vi "KE6485GUI.panel.vi"() -> ()   [LabVIEW 2014, in "KE6485GUI.lvlib"]
doc: "example GUI for a class inherited from the DeviceBaseGUI\n\nauthor: Dietrich Beck, GSI\nlicense: GPL"
uses:
  KE6485GUI.lvlib
  CSlibraries-extern/DimLVEvent/DimIndicators/DimIndicators.numericType.ctl
  CSlibraries-extern/DimLVEvent/LVDimInterface/LVDimInterface.dim service type.ctl
  <vilib>/Utility/file.llb/Write To Spreadsheet File (DBL).vi
  CS_Core/CSSystem/CoreLib/CoreLib.byte array 2 string.vi
  CS_Core/CSSystem/CoreLib/CoreLib.lvlib
  CS_Core/CSObj/CSObj.lvlib
  CS_Core/GUIs/GOGUserGUIs/DeviceBaseGUI/DeviceBaseGUI.lvlib
  CSlibraries-extern/DimLVEvent/DimIndicators/DimIndicators.lvlib
  CS_Core/CSSystem/CSSystemLib/CSSystemLib.lvlib
  CS_Core/BaseProcess/BaseProcess.lvlib
  CSlibraries-extern/DimLVEvent/LVDimInterface/LVDimInterface.lvlib
panel:
  out "Remaning time":string
  out "running?":bool
  out "ActDimensions":i16
  out "SActStep":i32
  out "SNofSteps":i32
  out "ScanValuesArray":dbl[](array[numeric])
  out "ScanNamesArray":string[](array[string])
  out "size(s)":i32
  in  "Scanner_Finished":T1
  out "DIM Notifier loop":i32
  in  "Free Delay (s)":dbl=1.0
  in  "Data points":u32
  in  "Free Run?":bool
  in  "Save Path":path
  in  "Save button":bool
  in  "Clear Button":bool
  out "actPPG":string
  out "actScanner":string
  out "actSequencer":string
  in  "actValueLink":T1 caption="dic_service_numeric"
  out "Busy":bool
  out "Logger String":string
  out "Progress bar":u8(slide) scale=0.0..100.0
  in  "Stop Scan button":bool
  in  "Pause Scan button":bool
  in  "Start Scan button":bool
  in  "Configure Scan button":bool
  out "chart":cluster{dbl, "data":dbl}[](graph)
  out "loop counter":i32
  out "error out":errorcluster
  in  "error in (no error)":errorcluster
  in  "object ref":refnum<vi>
  # "Scan control"
  # "Plot control"
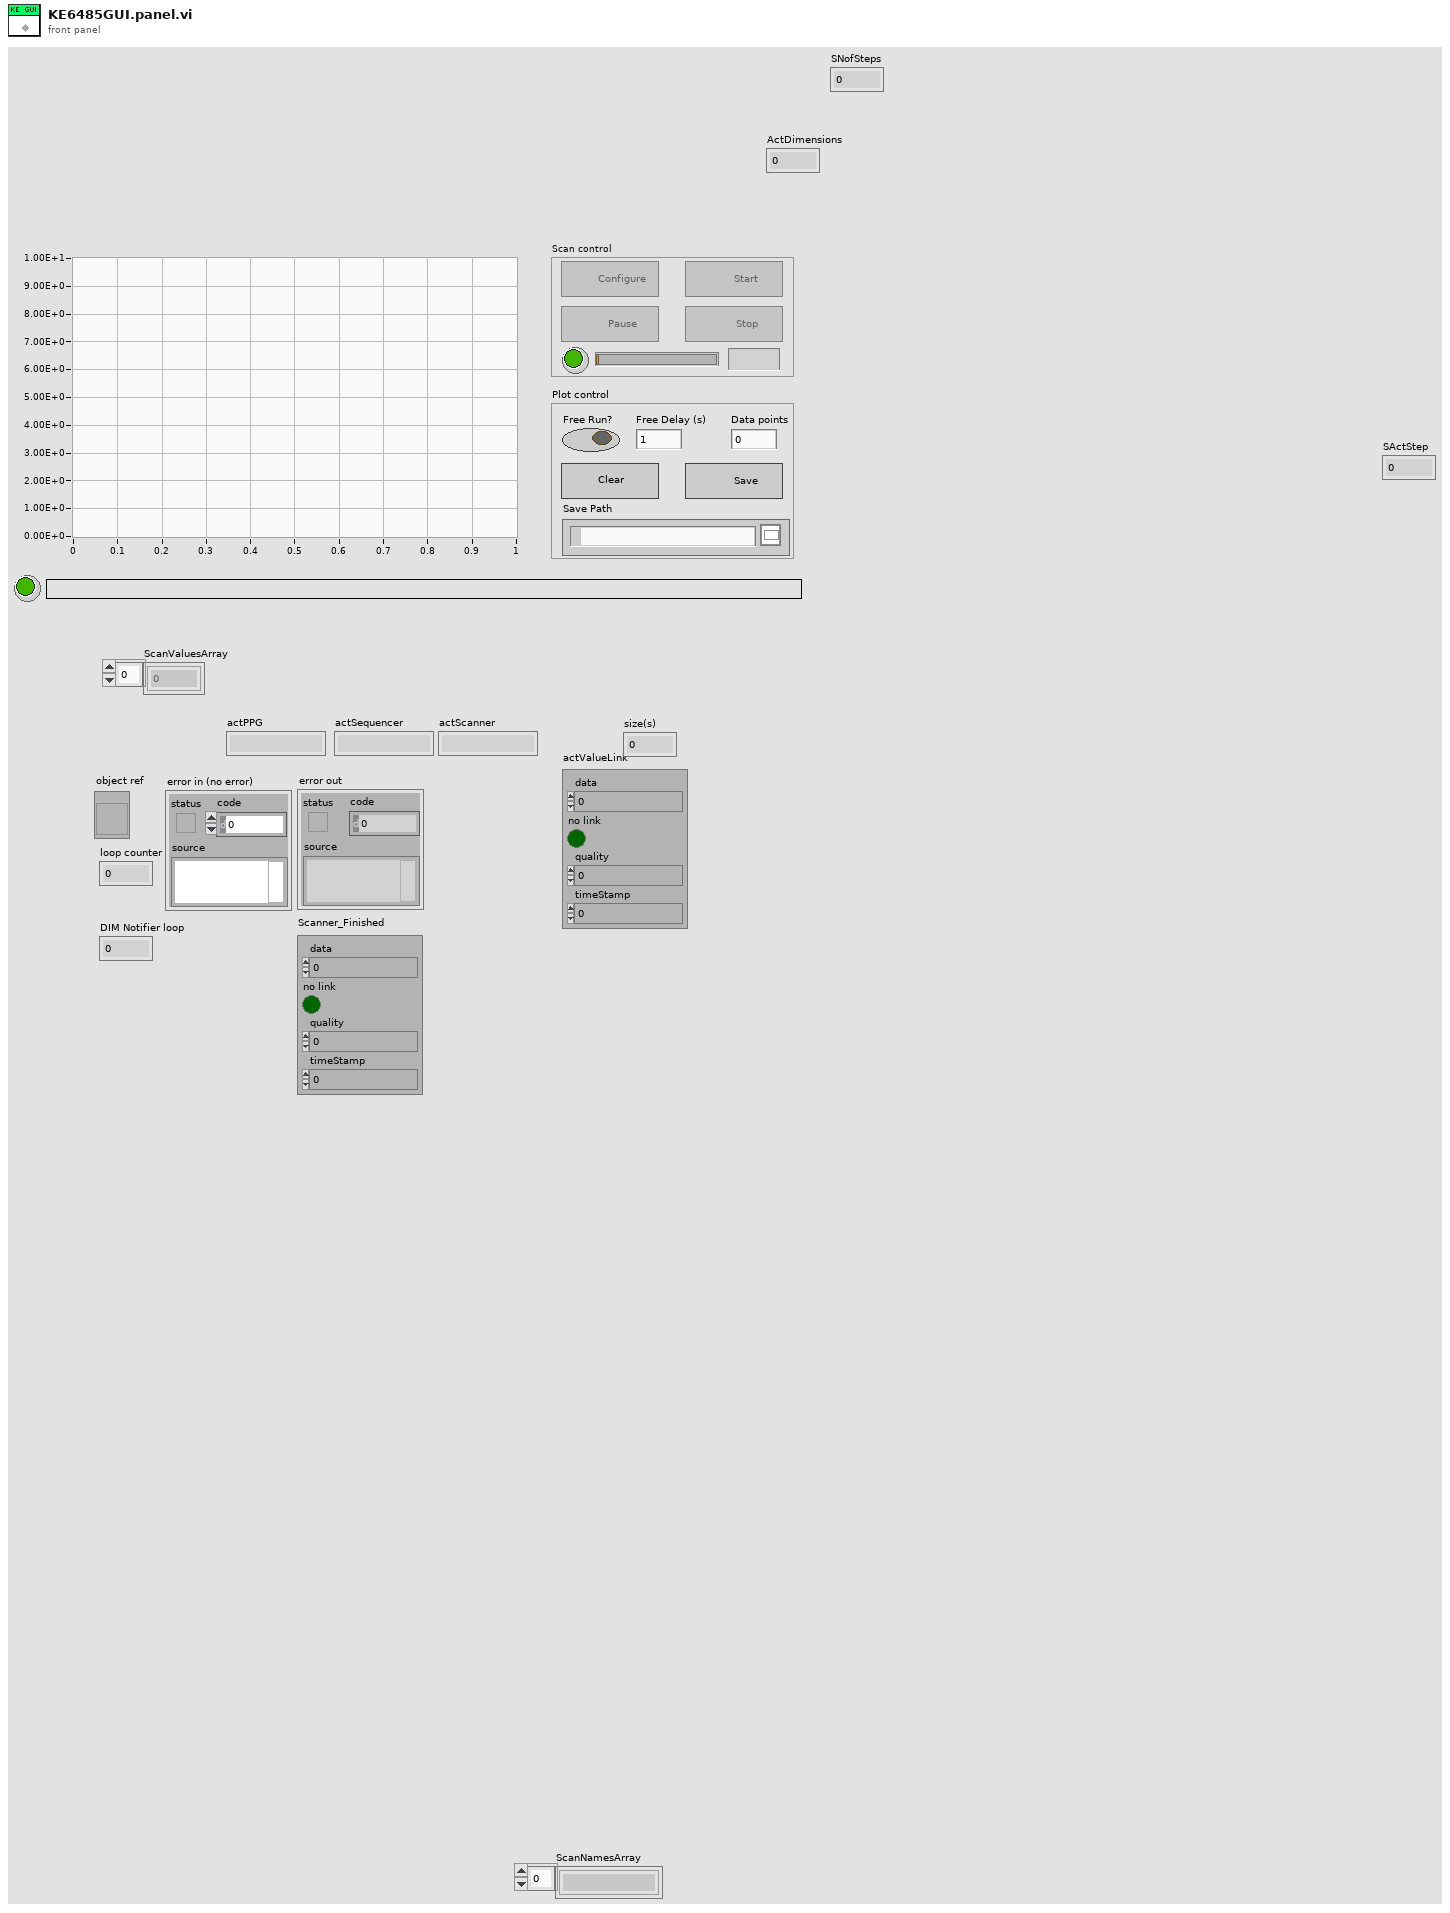
[diagram p1: front panel]
types:
  T1 = typedef "DimIndicators.lvlib/DimIndicators.numericType.ctl" = cluster{"data":dbl, "no link":bool, "quality":i32, "timeStamp":dbl}
  T2 = typedef "DeviceBaseGUI.lvlib/DeviceBaseGUI.i attribute.ctl" = cluster{"GOGFrontPanel.i attribute":T3}
  T3 = typedef "GOGFrontPanel.lvlib/GOGFrontPanel.i attribute.ctl" = cluster{"GOGObject":string, "Object":string, "Method":string, "Descriptor":T4, "Input Descriptor":string, "Output Descriptor":string, "inputNames":string[], "outputNames":string[], "Values":cluster{"descriptor":string, "value":string}[]}
  T4 = typedef "BaseProcess.lvlib/BaseProcess.descriptor string definition.ctl" = string
  T5 = enum8{"Enabled", "Disabled", "Disabled and Grayed Out"}
  T6 = typedef "CoreDefs.call_type.ctl" = cluster{"Object":string, "Selector":string, "CallType":enum16{"simple", "synchronous", "asynchronous"}, "Async Object":string, "Async Selector":string, "Data Descriptor":T4, "Data":T7, "Error #":i32, "Expire":u32}
  T7 = typedef "CoreDefs.rawDataType.ctl" = i8[]
  T8 = typedef "LVDimInterface.lvlib/LVDimInterface.dim service type.ctl" = u16
  T9 = typedef "LVRangeTypeDef.ctl" = cluster{"Minimum":dbl, "Maximum":dbl, "Increment":dbl, "Minor Increment":dbl, "Start":dbl}
  T10 = typedef "KE6485GUI.lvlib/KE6485GUI.i attribute.ctl" = cluster{"commandID":i32, "command notifier":refnum<notifier>}
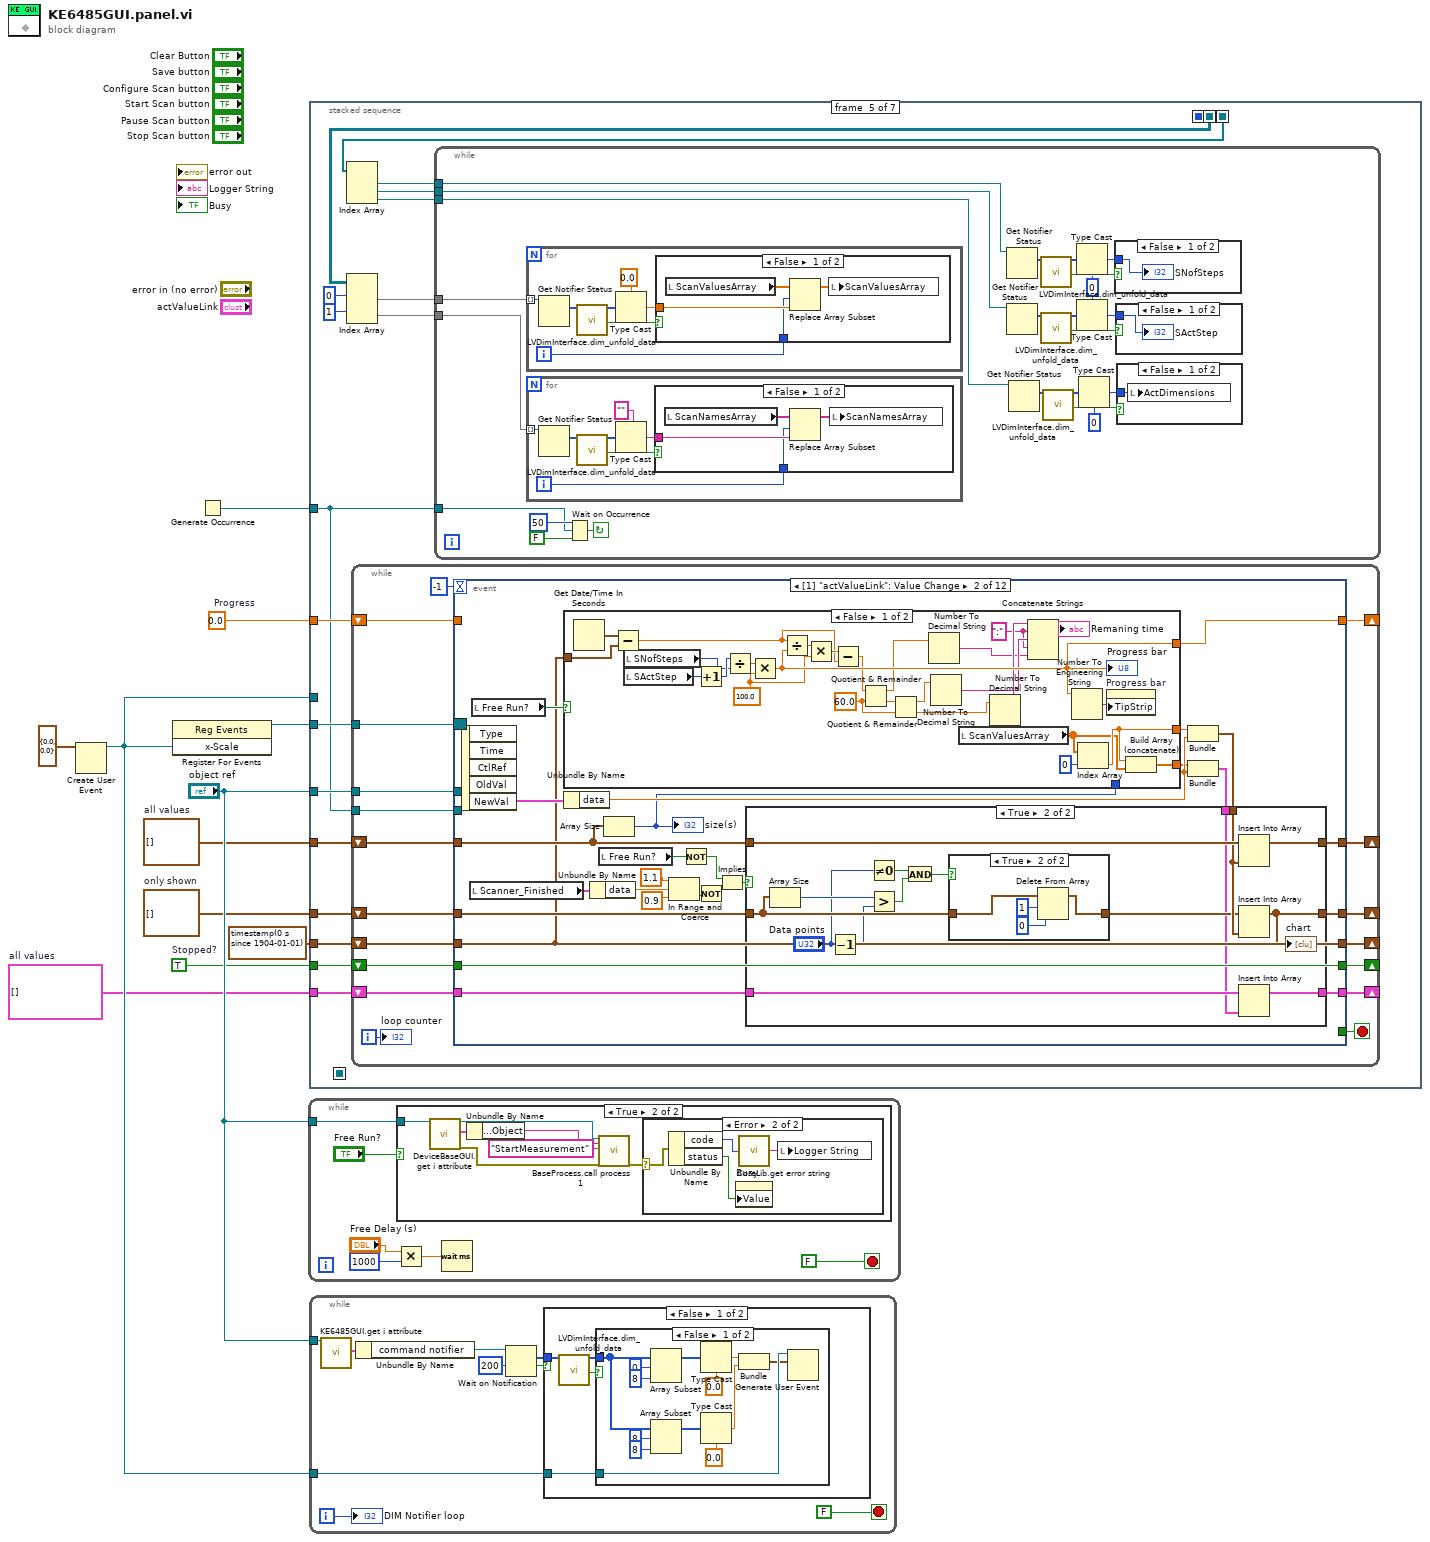
[diagram p0: block diagram]
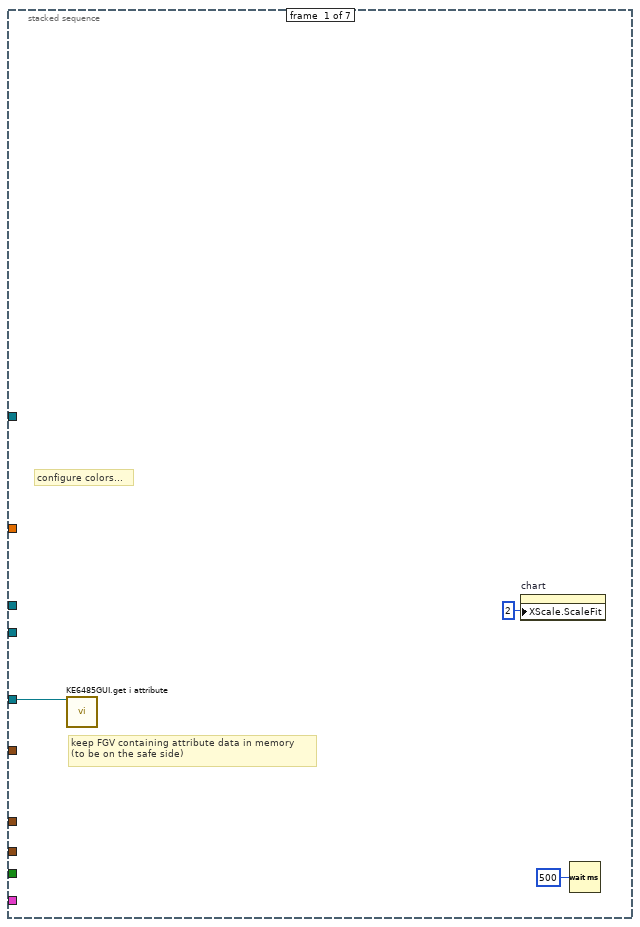
[diagram p6: hidden frame]
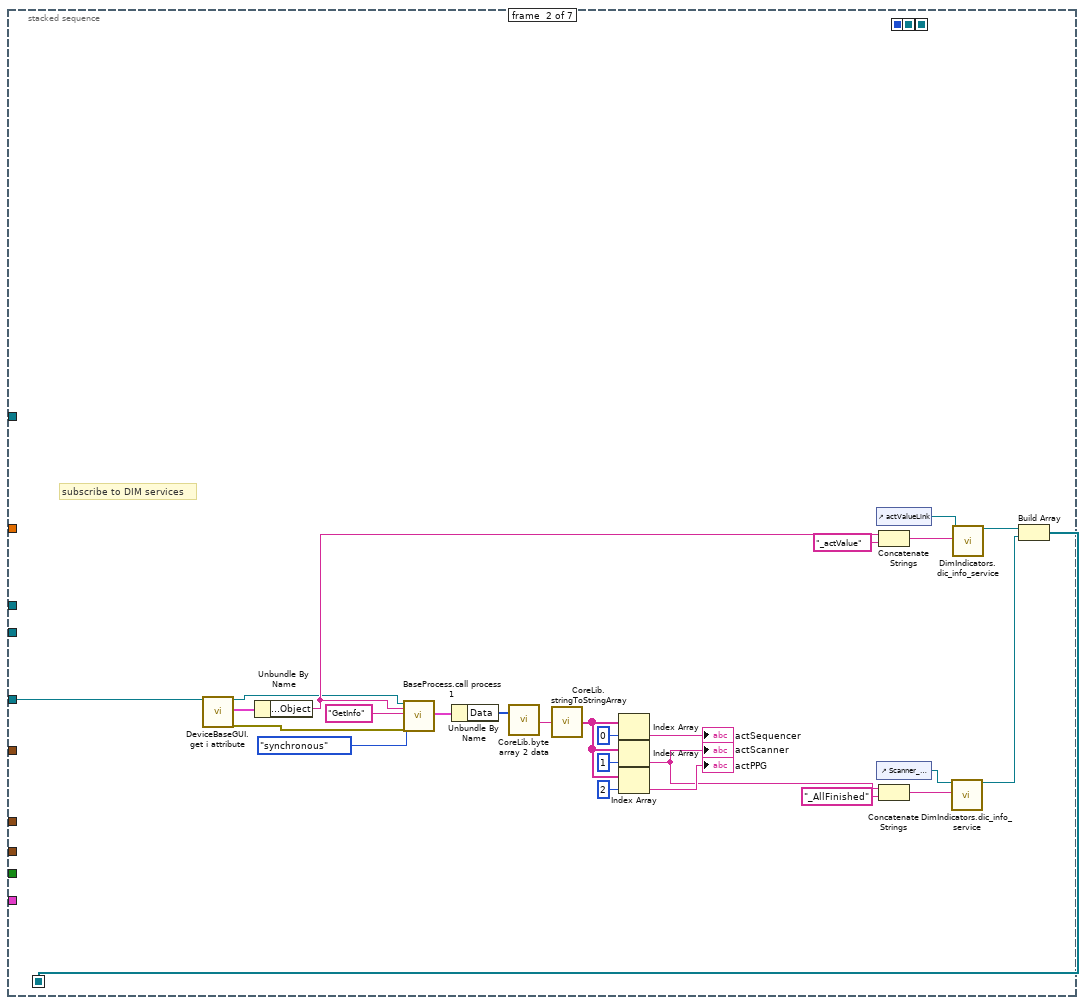
[diagram p7: hidden frame]
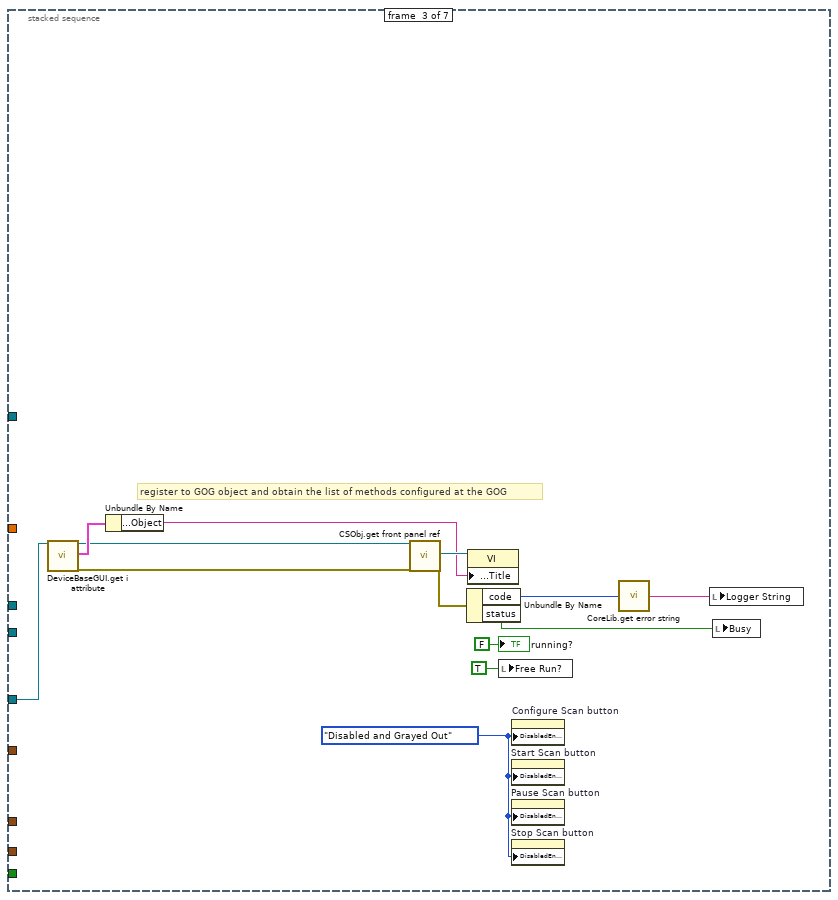
[diagram p8: hidden frame]
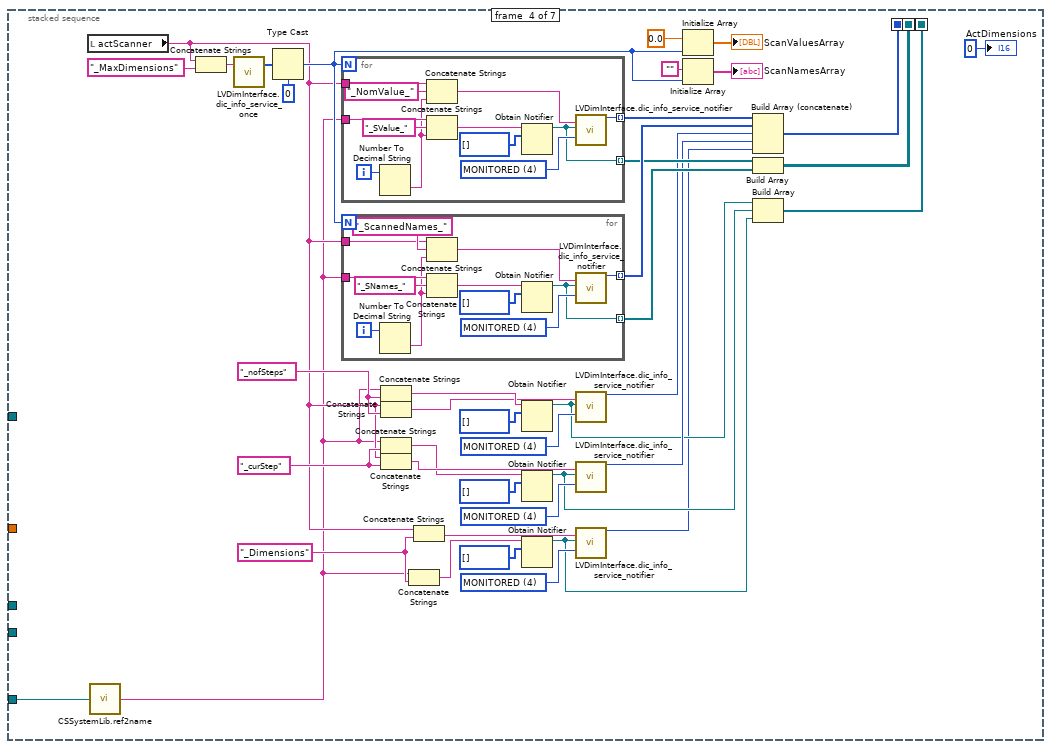
[diagram p9: hidden frame]
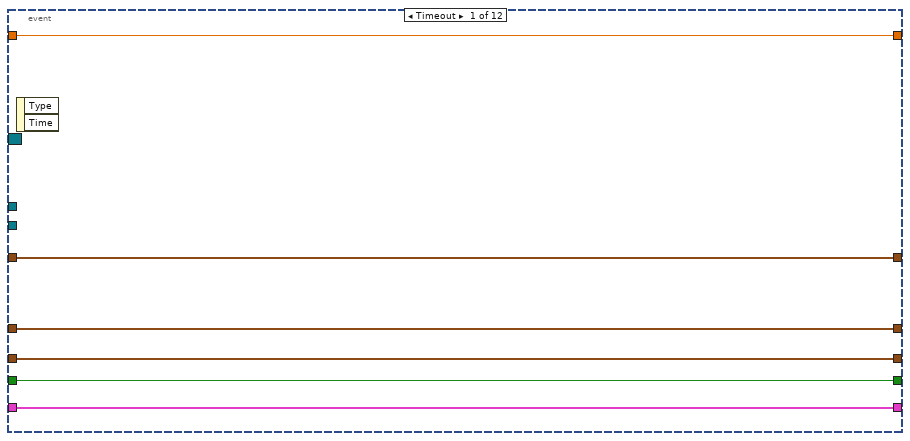
[diagram p15: hidden frame]
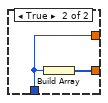
[diagram p18: hidden frame]
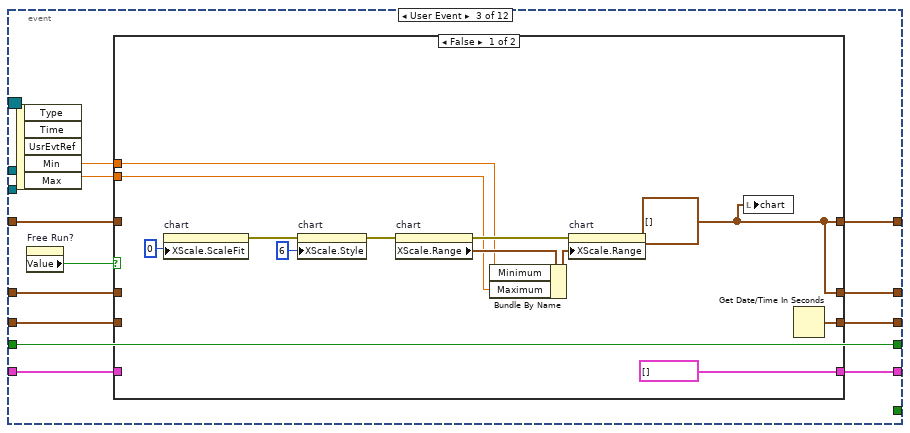
[diagram p19: hidden frame]
diagram:
  w3 = TRUE  # Stopped?
  w5 = 0.0  # Progress
  w6 = cluster{dbl, "data":dbl}[] []  # only shown
  w7 = cluster{dbl, "data":dbl}[] []  # all values
  w4 = cluster{"x-Values":dbl[], "y-Value":dbl}[] []  # all values
  n1 = Create User Event(user event datatype=cluster{"Min":dbl, "Max":dbl} {"Min"=0.0, "Max"=0.0} ("x-Scale")) -> (user event=w8:refnum<user-event>)  [unwired: 1 in, 1 out]
  n2 = register-events(w8) -> (reference out=w9:refnum<event-registration>)  [unwired: 2 in, 1 out]
  n3 = Generate Occurrence() -> (w2:refnum<k4>)
  n4 = while {
    tunnel: "object ref" -> [w16]
    stop <- FALSE stop-if-true
    n5 = Multiply(x="Free Delay (s)", y=u32 1000 ("milliseconds to wait")) -> (x*y=w12:dbl)
    n6 = case shown="True" "Free Run?" {
      tunnel: w16 -> [_ w24]
      frame False {
      }
      frame True {
        n7 = call "DeviceBaseGUI.get i attribute.vi"("i ref in"=w24) -> ("i ref out"=w21:refnum<vi>, "i attribute"=w23:T2, "error out"=w19:errorcluster)  [unwired: 16 in]
        n8 = Unbundle By Name(w23) -> ("GOGFrontPanel.i attribute.Object"=w22:string)
        n9 = call "BaseProcess.call process 1.vi"("i ref in"=w21, "Object"=w22, "Selector"="StartMeasurement", "error in (no error)"=w19) -> ("error out"=w18:errorcluster)  [unwired: 13 in, 2 out]
        n10 = case shown="Error" w18 {
          selector: w18 -> [_ w28]
          frame No Error {
          }
          frame Error {
            n11 = Unbundle By Name(w28) -> ("code"=w27:i32, "status"=w25:bool)
            n12 = property on="Busy" class="Bool (strict)"("Value"=w25) -> ()  [unwired: 2 in, 2 out]
            n13 = call "CoreLib.get error string.vi"("Error Code"=w27) -> ("Error String"=w26:string)
            n14 = local write "Logger String"(w26) -> ()
          }
        }
      }
    }
    n15 = Wait (ms)(milliseconds to wait=w12) -> ()  [unwired: 1 out]
  }
  n16 = stacked-sequence {
    seq-local: [_ w55 _ _ _ _ _] -> [_ _ _ _ _ w471 _]
    seq-local: [_ _ _ w97 _ _ _] -> [_ _ _ _ _ w469 _]
    seq-local: [_ _ _ w96 _ _ _] -> [_ _ _ _ w145 w467 _]
    seq-local: [_ _ _ w81 _ _ _] -> [_ _ _ _ w140 w468 _]
    tunnel: "object ref" -> [w30 w57 w70 w103 w153 _ w477]
    tunnel: w9 -> [_ _ _ _ w152 w470 _]
    tunnel: w8 -> [_ _ _ _ _ _ w476]
    tunnel: w7 -> [_ _ _ _ w151 _ _]
    tunnel: w6 -> [_ _ _ _ w150 _ _]
    tunnel: w5 -> [_ _ _ _ w149 _ _]
    tunnel: w4 -> [_ _ _ _ w148 _ _]
    tunnel: w3 -> [_ _ _ _ w147 _ _]
    tunnel: w2 -> [_ _ _ _ w146 _ _]
    tunnel: timestamp(0 s since 1904-01-01) ("seconds since 1Jan1904") -> [_ _ _ _ w136 _ _]
    frame #0 {
      # "keep FGV containing attribute data in memory\n(to be on the safe side)"
      # "configure colors..."
      n17 = call "KE6485GUI.get i attribute.vi"("i ref in"=w30) -> ()  [unwired: 16 in, 3 out]
      n18 = property on="chart" class="XYGraph (strict)"("XScale.ScaleFit"=u8 2 ("X Scale.Scale Fit")) -> ()  [unwired: 2 in, 2 out]
      n19 = Wait (ms)(milliseconds to wait=u32 500) -> ()  [unwired: 1 out]
    }
    frame #1 {
      # "subscribe to DIM services"
      n20 = call "DeviceBaseGUI.get i attribute.vi"("i ref in"=w57) -> ("i ref out"=w48:refnum<vi>, "i attribute"=w56:T2, "error out"=w47:errorcluster)  [unwired: 16 in]
      n21 = Unbundle By Name(w56) -> ("GOGFrontPanel.i attribute.Object"=w49:string)
      n22 = call "BaseProcess.call process 1.vi"("i ref in"=w48, "Object"=w49, "Selector"="GetInfo", "CallType"=enum16{"simple", "synchronous", "asynchronous"}."synchronous", "error in (no error)"=w47) -> ("call cluster out"=w46:T6)  [unwired: 12 in, 2 out]
      n23 = Unbundle By Name(w46) -> ("Data"=w45:T7)
      n24 = call-poly "CoreLib.byte array 2 data.vi"("byteArray"=w45) -> ("string"=w44:string)  [unwired: 16 in, 2 out]
      n25 = call "CoreLib.stringToStringArray.vi"("String"=w44) -> ("Array"=w43:string[])
      n26 = Index Array(array=w43, index=0) -> (element=→"actSequencer":string)
      n27 = Index Array(array=w43, index=1) -> (element=w33:string)
      "actScanner" <- w33
      n28 = Index Array(array=w43, index=2) -> (element=→"actPPG":string)
      n29 = control-ref of="actValueLink"() -> (w53:refnum<vi>)
      n30 = control-ref of="Scanner_Finished"() -> (w34:refnum<vi>)
      n31 = Concatenate Strings(w49, "_actValue" ("string")) -> (w54:string)
      n32 = Concatenate Strings(w33, "_AllFinished" ("string")) -> (w35:string)
      n33 = call "DimIndicators.dic_info_service.vi"("controlRef"=w34, "serviceName"=w35) -> ("controlRef out"=w32:refnum<vi>)  [unwired: 16 in, 1 out]
      n34 = call "DimIndicators.dic_info_service.vi"("controlRef"=w53, "serviceName"=w54) -> ("controlRef out"=w52:refnum<vi>)  [unwired: 16 in, 1 out]
      n35 = Build Array(w52, w32) -> (w55:refnum<vi>[])
    }
    frame #2 {
      w61 = T5."Disabled and Grayed Out" ("Disabled")
      # "register to GOG object and obtain the list of methods configured at the GOG"
      n36 = call "DeviceBaseGUI.get i attribute.vi"("i ref in"=w70) -> ("i ref out"=w60:refnum<vi>, "i attribute"=w69:T2, "error out"=w59:errorcluster)  [unwired: 16 in]
      n37 = Unbundle By Name(w69) -> ("GOGFrontPanel.i attribute.Object"=w67:string)
      n38 = call "CSObj.get front panel ref.vi"("i ref in"=w60, "error in (no error)"=w59) -> ("frontPanelRef"=w68:refnum<vi>, "error out"=w64:errorcluster)  [unwired: 15 in, 1 out]
      n39 = Unbundle By Name(w64) -> ("code"=w66:i32, "status"=w65:bool)
      n40 = property class="VI"(reference=w68, "Front Panel Window:Title"=w67) -> ()  [unwired: 1 in, 2 out]
      n41 = local write "Free Run?"(TRUE ("Free Run?")) -> ()
      n42 = property on="Configure Scan button" class="Bool"("DisabledEnum"=w61) -> ()  [unwired: 2 in, 2 out]
      n43 = property on="Start Scan button" class="Bool"("DisabledEnum"=w61) -> ()  [unwired: 2 in, 2 out]
      n44 = property on="Pause Scan button" class="Bool"("DisabledEnum"=w61) -> ()  [unwired: 2 in, 2 out]
      n45 = property on="Stop Scan button" class="Bool"("DisabledEnum"=w61) -> ()  [unwired: 2 in, 2 out]
      n46 = call "CoreLib.get error string.vi"("Error Code"=w66) -> ("Error String"=w63:string)
      n47 = local write "Logger String"(w63) -> ()
      n48 = local write "Busy"(w65) -> ()
      "running?" <- FALSE ("running?")
    }
    frame #3 {
      w77 = "_Dimensions" ("string")
      w79 = T8 4 items=["ONCE_ONLY"=1, "TIMED"=2, "MONITORED"=4] ("serviceType")
      w88 = T8 4 items=["ONCE_ONLY"=1, "TIMED"=2, "MONITORED"=4] ("serviceType")
      w93 = "_nofSteps" ("string")
      w92 = "_curStep" ("string")
      w94 = T8 4 items=["ONCE_ONLY"=1, "TIMED"=2, "MONITORED"=4] ("serviceType")
      n49 = local read "actScanner"() -> (w75:string)
      n50 = call "CSSystemLib.ref2name.vi"("obj refnum"=w103) -> ("name"=w74:string)
      n51 = Concatenate Strings(w75, "_MaxDimensions" ("string")) -> (w109:string)
      n52 = call "LVDimInterface.dic_info_service_once.vi"("serviceName"=w109) -> ("data"=w108:i8[])  [unwired: 15 in, 3 out]
      n53 = Type Cast(type=0, x=w108) -> (*(type *) &x=w111:i32)
      n54 = for {
        N: w111 -> [_]
        tunnel: w74 -> [w135]
        tunnel: w75 -> [w128]
        tunnel: [w125] -> w101 mode=indexing
        tunnel: [w124] -> w99 mode=indexing
        i -> [w133]
        w130 = T8 4 items=["ONCE_ONLY"=1, "TIMED"=2, "MONITORED"=4] ("serviceType")
        n55 = Number To Decimal String(number=w133) -> (decimal integer string=w127:string)  [unwired: 1 in]
        n56 = Concatenate Strings(w128, "_NomValue_", w127) -> (w126:string)
        n57 = Concatenate Strings(w135, "_SValue_" ("string"), w127) -> (w132:string)
        n58 = Obtain Notifier(name (unnamed)=w132, notification data type=i8[] []) -> (notifier out=w124:refnum<notifier>)  [unwired: 2 in, 2 out]
        n59 = call "LVDimInterface.dic_info_service_notifier.vi"("serviceName"=w126, "notifierRef"=w124, "serviceType"=w130) -> ("callBackID"=w125:i32)  [unwired: 15 in, 1 out]
      }
      n60 = for {
        N: w111 -> [_]
        tunnel: w74 -> [w123]
        tunnel: w75 -> [w116]
        tunnel: [w113] -> w100 mode=indexing
        tunnel: [w112] -> w98 mode=indexing
        i -> [w121]
        w118 = T8 4 items=["ONCE_ONLY"=1, "TIMED"=2, "MONITORED"=4] ("serviceType")
        n61 = Number To Decimal String(number=w121) -> (decimal integer string=w115:string)  [unwired: 1 in]
        n62 = Concatenate Strings(w116, "_ScannedNames_", w115) -> (w114:string)
        n63 = Concatenate Strings(w123, "_SNames_" ("string"), w115) -> (w120:string)
        n64 = Obtain Notifier(name (unnamed)=w120, notification data type=i8[] []) -> (notifier out=w112:refnum<notifier>)  [unwired: 2 in, 2 out]
        n65 = call "LVDimInterface.dic_info_service_notifier.vi"("serviceName"=w114, "notifierRef"=w112, "serviceType"=w118) -> ("callBackID"=w113:i32)  [unwired: 15 in, 1 out]
      }
      n66 = Concatenate Strings(w74, w93) -> (w91:string)
      n67 = Concatenate Strings(w75, w93) -> (w90:string)
      n68 = Concatenate Strings(w74, w92) -> (w86:string)
      n69 = Concatenate Strings(w75, w92) -> (w87:string)
      n70 = Concatenate Strings(w74, w77) -> (w76:string)
      n71 = Concatenate Strings(w75, w77) -> (w78:string)
      n72 = Obtain Notifier(name (unnamed)=w91, notification data type=i8[] []) -> (notifier out=w83:refnum<notifier>)  [unwired: 2 in, 2 out]
      n73 = Obtain Notifier(name (unnamed)=w86, notification data type=i8[] []) -> (notifier out=w82:refnum<notifier>)  [unwired: 2 in, 2 out]
      n74 = Obtain Notifier(name (unnamed)=w76, notification data type=i8[] []) -> (notifier out=w73:refnum<notifier>)  [unwired: 2 in, 2 out]
      n75 = call "LVDimInterface.dic_info_service_notifier.vi"("serviceName"=w90, "notifierRef"=w83, "serviceType"=w94) -> ("callBackID"=w85:i32)  [unwired: 15 in, 1 out]
      n76 = call "LVDimInterface.dic_info_service_notifier.vi"("serviceName"=w87, "notifierRef"=w82, "serviceType"=w88) -> ("callBackID"=w84:i32)  [unwired: 15 in, 1 out]
      n77 = call "LVDimInterface.dic_info_service_notifier.vi"("serviceName"=w78, "notifierRef"=w73, "serviceType"=w79) -> ("callBackID"=w72:i32)  [unwired: 15 in, 1 out]
      n78 = Initialize Array(0.0, w111) -> (→"ScanValuesArray":dbl[])
      n79 = Initialize Array("", w111) -> (→"ScanNamesArray":string[])
      n80 = Build Array (concatenate)(w101, w100, w85, w84, w72) -> (w97:i32[])
      n81 = Build Array(w99, w98) -> (w96:refnum<notifier>[][])
      n82 = Build Array(w83, w82, w73) -> (w81:refnum<notifier>[])
      "ActDimensions" <- i16 0 ("ActDimensions")
    }
    frame #4 {
      n83 = Index Array(array=w140) -> (element #1=w139:refnum<notifier>, element #2=w138:refnum<notifier>, element #3=w137:refnum<notifier>)  [unwired: 3 in]
      n84 = Index Array(array=w145, index (row) #1=0 ("index (row)"), index (row) #2=1 ("index (row)")) -> (element #1=w142:refnum<notifier>[], element #2=w141:refnum<notifier>[])  [unwired: 2 in]
      n85 = while {
        tunnel: w153 -> [w218]
        shift-right: [w215] -> _
        shift-left: w151 -> [w214]
        shift-right: [w212] -> _
        shift-left: w150 -> [w213]
        tunnel: w152 -> [w211]
        shift-right: [w209] -> _
        shift-left: w147 -> [w210]
        shift-right: [w207] -> _
        shift-left: w149 -> [w208]
        shift-right: [w205] -> _
        shift-left: w148 -> [w206]
        tunnel: w146 -> [w204]
        shift-right: [w202] -> _
        shift-left: w136 -> [w203]
        i -> [w219]
        stop <- w216 stop-if-true
        n86 = event shown="[1] \"actValueLink\": Value Change" {
          selector: w211 -> [_ _ _ _ _ _ _ _ _ _ _ _]
          dyn-events: _ -> [_ _ _ _ _ _ _ _ _ _ _ _]
          timeout: -1 -> [_ _ _ _ _ _ _ _ _ _ _ _]
          tunnel: w218 -> [_ _ _ _ w338 _ _ w403 _ w444 w456 _]
          tunnel: [_ _ _ _ _ _ _ _ _ _ _ w465] -> w216
          tunnel: [w225 w250 w315 w334 w340 w360 w371 w400 w419 w443 w454 w464] -> w215
          tunnel: w214 -> [w225 w233 w313 _ _ w360 w371 w399 w418 w443 _ w464]
          tunnel: w213 -> [w224 w248 w312 _ _ w358 w370 w397 w416 w442 _ w463]
          tunnel: [w224 w249 w314 w334 w340 w358 w370 w398 w417 w442 w454 w463] -> w212
          tunnel: w210 -> [w223 w247 w308 w333 _ w356 w369 w387 _ w438 _ w462]
          tunnel: [w223 w247 w308 w333 TRUE ("Stopped?") w356 w369 FALSE w415 w438 TRUE ("Stopped?") w462] -> w209
          tunnel: w208 -> [w222 _ _ _ _ w354 w368 w386 w414 w437 w450 w461]
          tunnel: [w222 w244 _ _ _ w354 w368 w385 w414 w437 w450 w461] -> w207
          tunnel: w206 -> [w221 w243 w307 _ _ w353 w367 w384 w412 w436 _ w460]
          tunnel: [w221 w242 w306 cluster{"x-Values":dbl[], "y-Value":dbl}[] [] ("all values") cluster{"x-Values":dbl[], "y-Value":dbl}[] [] ("all values") w353 w367 w383 w413 w436 cluster{"x-Values":dbl[], "y-Value":dbl}[] [] ("all values") w460] -> w205
          tunnel: w204 -> [_ _ _ _ _ _ _ _ _ _ _ w459]
          tunnel: w203 -> [w220 w226 w304 _ _ w352 w366 w381 w411 w434 w447 _]
          tunnel: [w220 w226 w305 _ _ w352 w366 w381 w411 w434 w447 _] -> w202
          event Timeout {
            n87 = event-data() -> ()  [unwired: 1 in, 2 out]
          }
          event Value Change {
            n88 = event-data() -> ("NewVal"=w251:T1)  [unwired: 1 in, 4 out]
            n89 = local read "Scanner_Finished"() -> (w234:T1)
            n90 = local read "Free Run?"() -> (w238:bool)
            n91 = Unbundle By Name(w251) -> ("data"=w240:dbl)
            n92 = Unbundle By Name(w234) -> ("data"=w237:dbl)
            n93 = local read "Free Run?"() -> (w230:bool)
            n94 = Array Size(array=w233) -> (size(s)=w232:i32)
            "size(s)" <- w232
            n95 = case shown="False" w238 {
              tunnel: [w294 w303] -> w245
              tunnel: w232 -> [_ w303]
              tunnel: [w290 _] -> w244
              tunnel: [w298 w302] -> w239
              tunnel: w226 -> [w291 _]
              frame False {
                w278 = ":" ("string")
                w284 = 60.0 ("y")
                w288 = 100.0 ("y")
                n96 = Get Date/Time In Seconds() -> (seconds since 1Jan1904=w292:timestamp)
                n97 = Subtract(x=w292, y=w291) -> (x-y=w286:dbl)
                n98 = local read "SNofSteps"() -> (w296:i32)
                n99 = local read "SActStep"() -> (w297:i32)
                n100 = Increment(x=w297) -> (x+1=w300:i32)
                n101 = Divide(x=w300, y=w296) -> (x/y=w301:dbl)
                n102 = Multiply(x=w301, y=w288) -> (x*y=w290:dbl)
                "Progress bar" <- w290
                n103 = Divide(x=w286, y=w290) -> (x/y=w289:dbl)
                n104 = Multiply(x=w289, y=w288) -> (x*y=w287:dbl)
                n105 = Subtract(x=w287, y=w286) -> (x-y=w285:dbl)
                n106 = Quotient & Remainder(x=w285, y=w284) -> (x-y*floor(x/y)=w276:dbl, floor(x/y)=w283:dbl)
                n107 = Quotient & Remainder(x=w283, y=w284) -> (x-y*floor(x/y)=w275:dbl, floor(x/y)=w282:dbl)
                n108 = Number To Decimal String(number=w276) -> (decimal integer string=w277:string)  [unwired: 1 in]
                n109 = Number To Decimal String(number=w275) -> (decimal integer string=w279:string)  [unwired: 1 in]
                n110 = local read "ScanValuesArray"() -> (w293:dbl[])
                n111 = Number To Decimal String(number=w282) -> (decimal integer string=w280:string)  [unwired: 1 in]
                n112 = Concatenate Strings(w280, w278, w279, w278, w277) -> (→"Remaning time":string)
                n113 = Number To Engineering String(4:w290) -> (0:w299:string)  [unwired: 3 in]
                n114 = Index Array(array=w293, index=0) -> (element=w294:dbl)
                n115 = property on="Progress bar" class="Slide (strict)"("TipStrip"=w299) -> ()  [unwired: 2 in, 2 out]
                n116 = Build Array (concatenate)(w294, w293) -> (w298:dbl[])
              }
              frame True {
                n117 = Build Array(w303) -> (w302:i32[])
              }
            }
            n118 = In Range and Coerce(upper limit=1.1, x=w237, lower limit=0.9) -> (In Range?=w229:bool)  [unwired: 1 out]
            n119 = Not(x=w230) -> (.not. x?=w228:bool)
            n120 = Not(x=w229) -> (.not. x?=w227:bool)
            n121 = Implies(1:w227, 2:w228) -> (0:w231:bool)
            n122 = Bundle(w245, "data"=w240) -> (w246:cluster{dbl, "data":dbl})  [unwired: 1 in]
            n123 = Bundle(w239, "data"=w240) -> (w241:cluster{dbl[], "data":dbl})  [unwired: 1 in]
            n124 = case shown="True" w231 {
              tunnel: [w254 w269] -> w250
              tunnel: w233 -> [w254 w268]
              tunnel: [w253 w267] -> w249
              tunnel: w248 -> [w253 w266]
              tunnel: w246 -> [_ w265]
              tunnel: w243 -> [w252 w257]
              tunnel: [w252 w256] -> w242
              tunnel: w241 -> [_ w255]
              frame False {
              }
              frame True {
                n125 = Array Size(array=w266) -> (size(s)=w264:i32)
                n126 = Decrement(x="Data points") -> (x-1=w259:u32)
                n127 = Not Equal To 0?(x="Data points") -> (x != 0?=w263:bool)
                n128 = Greater?(x=w264, y=w259) -> (0:w262:bool)
                n129 = And(x=w263, y=w262) -> (x .and. y?=w261:bool)
                n130 = case shown="True" w261 {
                  tunnel: w266 -> [w270 w274]
                  tunnel: [w270 w273] -> w260
                  frame False {
                  }
                  frame True {
                    n131 = Delete From Array(array=w274, length=1, index=0) -> (array with subset deleted=w273:cluster{dbl, "data":dbl}[])  [unwired: 1 out]
                  }
                }
                n132 = Insert Into Array(array=w268, new element=w265) -> (w269:cluster{dbl, "data":dbl}[])  [unwired: 1 in]
                n133 = Insert Into Array(array=w260, new element=w265) -> (w267:cluster{dbl, "data":dbl}[])  [unwired: 1 in]
                "chart" <- w267
                n134 = Insert Into Array(array=w257, new element=w255) -> (w256:cluster{"x-Values":dbl[], "y-Value":dbl}[])  [unwired: 1 in]
              }
            }
          }
          event User Event {
            n135 = event-data() -> ("Min"=w310:dbl, "Max"=w309:dbl)  [unwired: 1 in, 3 out]
            n136 = property on="Free Run?" class="Bool (strict)"() -> ("Value"=w311:bool)  [unwired: 2 in, 2 out]
            n137 = case shown="False" w311 {
              tunnel: [w321 w331] -> w315
              tunnel: [w321 w330] -> w314
              tunnel: w313 -> [_ w331]
              tunnel: w312 -> [_ w330]
              tunnel: w310 -> [w323 _]
              tunnel: w309 -> [w322 _]
              tunnel: w307 -> [_ w329]
              tunnel: [cluster{"x-Values":dbl[], "y-Value":dbl}[] [] ("all values") w329] -> w306
              tunnel: [w316 w328] -> w305
              tunnel: w304 -> [_ w328]
              frame False {
                w321 = cluster{dbl, "data":dbl}[] []
                n138 = property on="chart" class="XYGraph (strict)"("XScale.ScaleFit"=u8 0 ("X Scale.Scale Fit")) -> (error out=w319:errorcluster)  [unwired: 2 in, 1 out]
                n139 = property on="chart" class="XYGraph (strict)"(error in=w319, "XScale.Style"=u8 6 ("X Scale.Style")) -> (error out=w318:errorcluster)  [unwired: 1 in, 1 out]
                n140 = property on="chart" class="XYGraph (strict)"(error in=w318) -> (error out=w326:errorcluster, "XScale.Range"=w325:T9)  [unwired: 1 in, 1 out]
                n141 = Bundle By Name(cluster=w325, "Minimum"=w323, "Maximum"=w322) -> (w324:T9)
                n142 = property on="chart" class="XYGraph (strict)"(error in=w326, "XScale.Range"=w324) -> ()  [unwired: 1 in, 2 out]
                n143 = local write "chart"(w321) -> ()
                n144 = Get Date/Time In Seconds() -> (seconds since 1Jan1904=w316:timestamp)
              }
              frame True {
              }
            }
          }
          event "Clear Button": Value Change {
            w334 = cluster{dbl, "data":dbl}[] []
            n145 = event-data() -> ()  [unwired: 1 in, 5 out]
            n146 = invoke on="chart" class="XYGraph (strict)" method="Reinit To Default"() -> ()  [unwired: 3 in, 3 out]
            n147 = invoke on="Clear Button" class="Bool" method="Reinit To Default"() -> ()  [unwired: 3 in, 3 out]
          }
          event "Free Run?": Value Change {
            w340 = cluster{dbl, "data":dbl}[] []  # all values
            n148 = event-data() -> ("NewVal"=w341:bool)  [unwired: 1 in, 4 out]
            n149 = case shown="True" w341 {
              tunnel: [T5."Enabled" ("Disabled") w349] -> w342
              tunnel: [w343 T5."Enabled" ("Disabled")] -> w336
              tunnel: [w343 w349] -> w339
              tunnel: w338 -> [_ w347]
              frame False {
                w343 = T5."Disabled and Grayed Out" ("Disabled")
              }
              frame True {
                w349 = T5."Disabled and Grayed Out" ("Disabled")
                n150 = invoke on="chart" class="XYGraph (strict)" method="Reinit To Default"() -> (error out=w345:errorcluster)  [unwired: 3 in, 2 out]
                n151 = local read "actSequencer"() -> (w346:string)
                n152 = property on="chart" class="XYGraph (strict)"(error in=w345, "XScale.ScaleFit"=u8 2 ("X Scale.Scale Fit")) -> ()  [unwired: 1 in, 2 out]
                n153 = call "BaseProcess.call process 2.vi"("i ref in"=w347, "Object"=w346, "Selector"="Abort") -> ()  [unwired: 15 in, 2 out]
              }
            }
            n154 = property on="Configure Scan button" class="Bool"("DisabledEnum"=w342) -> ()  [unwired: 2 in, 2 out]
            n155 = property on="Start Scan button" class="Bool"("DisabledEnum"=w342) -> ()  [unwired: 2 in, 2 out]
            n156 = property on="Pause Scan button" class="Bool"("DisabledEnum"=w339) -> ()  [unwired: 2 in, 2 out]
            n157 = property on="Stop Scan button" class="Bool"("DisabledEnum"=w339) -> ()  [unwired: 2 in, 2 out]
            n158 = property on="Free Delay (s)" class="DigNum (strict)"("DisabledEnum"=w336) -> ()  [unwired: 2 in, 2 out]
            n159 = property on="Data points" class="DigNum (strict)"("DisabledEnum"=w336) -> ()  [unwired: 2 in, 2 out]
          }
          event "Save button": Value Change {
            n160 = event-data() -> ()  [unwired: 1 in, 5 out]
            n161 = for {
              tunnel: w353 -> [w365] mode=indexing
              tunnel: [w362] -> w357 mode=indexing
              n162 = Unbundle(w365) -> ("x-Values"=w364:dbl[], "y-Value"=w363:dbl)
              n163 = Build Array (concatenate)(w364, w363) -> (w362:dbl[])
            }
            n164 = invoke on="Save button" class="Bool" method="Reinit To Default"() -> ()  [unwired: 3 in, 3 out]
            n165 = call-poly <vilib>:"Write To Spreadsheet File.vi"("format (%.3f)"="%.6f", "append to file? (new file:F)"=FALSE, "2D data"=w357, "file path (dialog if empty)"="Save Path") -> ()  [unwired: 4 in, 1 out]
          }
          event "Configure Scan button": Value Change {
            n166 = event-data() -> ()  [unwired: 1 in, 5 out]
            n167 = invoke on="Configure Scan button" class="Bool" method="Reinit To Default"() -> ()  [unwired: 3 in, 3 out]
            n168 = local read "actSequencer"() -> (w378:string)
            n169 = local read "actPPG"() -> (w372:string)
            n170 = call "CSSystemLib.name2ref.vi"("name"=w378) -> ("obj refnum"=w380:refnum<vi>)
            n171 = call "CSSystemLib.name2ref.vi"("name"=w372) -> ("obj refnum"=w374:refnum<vi>)
            n172 = call "CSObj.open front panel.vi"("i ref in"=w380, "frontPanelOpen"=TRUE ("front panel open")) -> ()  [unwired: 16 in, 2 out]
            n173 = local read "actScanner"() -> (w375:string)
            n174 = call "CSObj.open front panel.vi"("i ref in"=w374, "frontPanelOpen"=TRUE ("front panel open")) -> ()  [unwired: 16 in, 2 out]
            n175 = call "CSSystemLib.name2ref.vi"("name"=w375) -> ("obj refnum"=w377:refnum<vi>)
            n176 = call "CSObj.open front panel.vi"("i ref in"=w377, "frontPanelOpen"=TRUE ("front panel open")) -> ()  [unwired: 16 in, 2 out]
          }
          event "Start Scan button": Value Change {
            w391 = T5."Enabled" ("Disabled")
            # "Start button to use after scan has stopped automatically AND after Pause was pressed"
            n177 = event-data() -> ()  [unwired: 1 in, 5 out]
            n178 = Unbundle By Name("Scanner_Finished") -> ("data"=w395:dbl)
            n179 = In Range and Coerce(upper limit=1.1, x=w395, lower limit=0.9) -> (In Range?=w390:bool)  [unwired: 1 out]
            n180 = property on="Start Scan button" class="Bool"("DisabledEnum"=T5."Disabled and Grayed Out" ("Disabled")) -> ()  [unwired: 2 in, 2 out]
            n181 = property on="Pause Scan button" class="Bool"("DisabledEnum"=w391) -> ()  [unwired: 2 in, 2 out]
            n182 = property on="Stop Scan button" class="Bool"("DisabledEnum"=w391) -> ()  [unwired: 2 in, 2 out]
            n183 = Or(x=w390, y=w387) -> (x .or. y?=w389:bool)
            n184 = case shown="True" w389 {
              tunnel: [w408 w410] -> w400
              tunnel: w399 -> [w408 _]
              tunnel: [w407 w410] -> w398
              tunnel: w397 -> [w407 _]
              tunnel: w386 -> [w406 _]
              tunnel: [w406 _] -> w385
              tunnel: w384 -> [w405 _]
              tunnel: [w405 cluster{"x-Values":dbl[], "y-Value":dbl}[] [] ("all values")] -> w383
              frame False {
              }
              frame True {
                w410 = cluster{dbl, "data":dbl}[] []  # all values
              }
            }
            n185 = local write "running?"(TRUE ("running?")) -> ()
            n186 = invoke on="Start Scan button" class="Bool" method="Reinit To Default"() -> (error out=w401:errorcluster)  [unwired: 3 in, 2 out]
            n187 = local read "actSequencer"() -> (w402:string)
            n188 = call "BaseProcess.call process 2.vi"("i ref in"=w403, "Object"=w402, "Selector"="Start", "error in (no error)"=w401) -> ()  [unwired: 14 in, 2 out]
          }
          event Value Change {
            n189 = event-data() -> ("NewVal"=w420:dbl)  [unwired: 1 in, 4 out]
            n190 = In Range and Coerce(upper limit=1.1, x=w420, lower limit=0.9) -> (In Range?=w421:bool)  [unwired: 1 out]
            n191 = case shown="True" w421 {
              tunnel: [w426 w431] -> w419
              tunnel: w418 -> [w426 w431]
              tunnel: [w425 w430] -> w417
              tunnel: w416 -> [w425 w430]
              tunnel: [_ TRUE] -> w415
              tunnel: [w424 w428] -> w413
              tunnel: w412 -> [w424 w428]
              frame False {
              }
              frame True {
                w432 = T5."Disabled and Grayed Out" ("Disabled")
                n192 = local write "running?"(FALSE ("running?")) -> ()
                n193 = property on="Start Scan button" class="Bool"("DisabledEnum"=T5."Enabled" ("Disabled")) -> ()  [unwired: 2 in, 2 out]
                n194 = property on="Stop Scan button" class="Bool"("DisabledEnum"=w432) -> ()  [unwired: 2 in, 2 out]
                n195 = property on="Pause Scan button" class="Bool"("DisabledEnum"=w432) -> ()  [unwired: 2 in, 2 out]
              }
            }
          }
          event "Pause Scan button": Value Change {
            n196 = event-data() -> ()  [unwired: 1 in, 5 out]
            n197 = invoke on="Pause Scan button" class="Bool" method="Reinit To Default"() -> ()  [unwired: 3 in, 3 out]
            n198 = local write "running?"(FALSE ("running?")) -> ()
            n199 = local read "actSequencer"() -> (w445:string)
            n200 = call "BaseProcess.call process 2.vi"("i ref in"=w444, "Object"=w445, "Selector"="Pause") -> ()  [unwired: 15 in, 2 out]
            n201 = property on="Start Scan button" class="Bool"("DisabledEnum"=T5."Enabled" ("Disabled")) -> ()  [unwired: 2 in, 2 out]
            n202 = property on="Pause Scan button" class="Bool"("DisabledEnum"=T5."Disabled and Grayed Out" ("Disabled")) -> ()  [unwired: 2 in, 2 out]
            n203 = property on="Stop Scan button" class="Bool"("DisabledEnum"=T5."Enabled" ("Disabled")) -> ()  [unwired: 2 in, 2 out]
          }
          event "Stop Scan button": Value Change {
            w452 = T5."Disabled and Grayed Out" ("Disabled")
            w454 = cluster{dbl, "data":dbl}[] []  # all values
            n204 = event-data() -> ()  [unwired: 1 in, 5 out]
            n205 = invoke on="Stop Scan button" class="Bool" method="Reinit To Default"() -> (error out=w455:errorcluster)  [unwired: 3 in, 2 out]
            n206 = local write "running?"(FALSE ("running?")) -> ()
            n207 = local read "actSequencer"() -> (w457:string)
            n208 = call "BaseProcess.call process 2.vi"("i ref in"=w456, "Object"=w457, "Selector"="Abort", "error in (no error)"=w455) -> ()  [unwired: 14 in, 2 out]
            n209 = property on="Start Scan button" class="Bool"("DisabledEnum"=T5."Enabled" ("Disabled")) -> ()  [unwired: 2 in, 2 out]
            n210 = property on="Pause Scan button" class="Bool"("DisabledEnum"=w452) -> ()  [unwired: 2 in, 2 out]
            n211 = property on="Stop Scan button" class="Bool"("DisabledEnum"=w452) -> ()  [unwired: 2 in, 2 out]
          }
          event Panel Close? {
            w465 = TRUE ("Discard?")
            n212 = event-data() -> ()  [unwired: 1 in, 4 out]
            n213 = Set Occurrence(w459) -> ()
            n214 = event-data("Discard?"=w465) -> ()  [unwired: 1 in, 1 out]
          }
        }
        "loop counter" <- w219
      }
      n215 = while {
        tunnel: w146 -> [w173]
        tunnel: w142 -> [w172]
        tunnel: w141 -> [w171]
        tunnel: w139 -> [w161]
        tunnel: w138 -> [w160]
        tunnel: w137 -> [w154]
        stop <- w174 continue-if-true
        w164 = 0
        n216 = for {
          tunnel: w172 -> [w195] mode=indexing
          i -> [w191]
          n217 = Get Notifier Status(notifier=w195) -> (current notification=w197:i8[])  [unwired: 1 in, 4 out]
          n218 = call "LVDimInterface.dim_unfold_data.vi"("rawData"=w197) -> ("data"=w196:i8[], "no link"=w194:bool)  [unwired: 15 in, 2 out]
          n219 = Type Cast(type=0.0, x=w196) -> (*(type *) &x=w192:dbl)
          n220 = case shown="False" w194 {
            tunnel: w192 -> [w199 _]
            tunnel: w191 -> [w198 _]
            frame False {
              n221 = local read "ScanValuesArray"() -> (w201:dbl[])
              n222 = Replace Array Subset(array=w201, new element=w199, index=w198) -> (w200:dbl[])
              n223 = local write "ScanValuesArray"(w200) -> ()
            }
            frame True {
            }
          }
        }
        n224 = for {
          tunnel: w171 -> [w184] mode=indexing
          i -> [w181]
          n225 = Get Notifier Status(notifier=w184) -> (current notification=w186:i8[])  [unwired: 1 in, 4 out]
          n226 = call "LVDimInterface.dim_unfold_data.vi"("rawData"=w186) -> ("data"=w185:i8[], "no link"=w183:bool)  [unwired: 15 in, 2 out]
          n227 = Type Cast(type="", x=w185) -> (*(type *) &x=w182:string)
          n228 = case shown="False" w183 {
            tunnel: w182 -> [w190 _]
            tunnel: w181 -> [w189 _]
            frame False {
              n229 = local read "ScanNamesArray"() -> (w188:string[])
              n230 = Replace Array Subset(array=w188, new element=w190, index=w189) -> (w187:string[])
              n231 = local write "ScanNamesArray"(w187) -> ()
            }
            frame True {
            }
          }
        }
        n232 = Wait on Occurrence(1:FALSE ("ignore previous (T)"), 2:w173, 3:50 ("ms timeout (-1)")) -> (0:w174:bool)
        n233 = Get Notifier Status(notifier=w161) -> (current notification=w170:i8[])  [unwired: 1 in, 4 out]
        n234 = Get Notifier Status(notifier=w160) -> (current notification=w165:i8[])  [unwired: 1 in, 4 out]
        n235 = Get Notifier Status(notifier=w154) -> (current notification=w159:i8[])  [unwired: 1 in, 4 out]
        n236 = call "LVDimInterface.dim_unfold_data.vi"("rawData"=w170) -> ("data"=w169:i8[], "no link"=w168:bool)  [unwired: 15 in, 2 out]
        n237 = call "LVDimInterface.dim_unfold_data.vi"("rawData"=w165) -> ("data"=w166:i8[], "no link"=w162:bool)  [unwired: 15 in, 2 out]
        n238 = call "LVDimInterface.dim_unfold_data.vi"("rawData"=w159) -> ("data"=w158:i8[], "no link"=w156:bool)  [unwired: 15 in, 2 out]
        n239 = Type Cast(type=w164, x=w169) -> (*(type *) &x=w167:i32)
        n240 = Type Cast(type=w164, x=w166) -> (*(type *) &x=w163:i32)
        n241 = Type Cast(type=i16 0, x=w158) -> (*(type *) &x=w155:i16)
        n242 = case shown="False" w168 {
          tunnel: w167 -> [w179 _]
          frame False {
            "SNofSteps" <- w179
          }
          frame True {
          }
        }
        n243 = case shown="False" w162 {
          tunnel: w163 -> [w178 _]
          frame False {
            "SActStep" <- w178
          }
          frame True {
          }
        }
        n244 = case shown="False" w156 {
          tunnel: w155 -> [w177 _]
          frame False {
            n245 = local write "ActDimensions"(w177) -> ()
          }
          frame True {
          }
        }
      }
    }
    frame #5 {
      n246 = Unregister For Events(event registration refnum=w470) -> ()  [unwired: 1 in, 1 out]
      n247 = for {
        tunnel: w471 -> [w475] mode=indexing
        n248 = call "DimIndicators.dic_release_service.vi"("controlRef"=w475) -> ()  [unwired: 18 in, 1 out]
      }
      n249 = Build Array (concatenate)(w468, w467) -> (w466:refnum<notifier>[][])
      n250 = for {
        tunnel: w466 -> [w472] mode=indexing
        n251 = for {
          tunnel: w472 -> [w473] mode=indexing
          n252 = Release Notifier(notifier=w473) -> ()  [unwired: 2 in, 3 out]
        }
      }
      n253 = for {
        tunnel: w469 -> [w474] mode=indexing
        n254 = call "LVDimInterface.dic_release_service.vi"("callBackID"=w474) -> ()  [unwired: 18 in, 1 out]
      }
    }
    frame #6 {
      n255 = Destroy User Event(user event=w476) -> ()  [unwired: 1 in, 1 out]
      n256 = call "DeviceBaseGUI.close panel.vi"("i ref in"=w477) -> ()  [unwired: 17 in, 2 out]
    }
  }
  n257 = while {
    tunnel: "object ref" -> [w484]
    tunnel: w8 -> [w479]
    i -> [w478]
    stop <- FALSE stop-if-true
    n258 = call "KE6485GUI.get i attribute.vi"("i ref in"=w484) -> ("i attribute"=w483:T10)  [unwired: 16 in, 2 out]
    n259 = Unbundle By Name(w483) -> ("command notifier"=w482:refnum<notifier>)
    n260 = Wait on Notification(notifier=w482, timeout in ms (-1)=200) -> (notification=w480:i8[], timed out?=w481:bool)  [unwired: 2 in, 2 out]
    n261 = case shown="False" w481 {
      tunnel: w480 -> [w490 _]
      tunnel: w479 -> [w487 _]
      frame False {
        n262 = call "LVDimInterface.dim_unfold_data.vi"("rawData"=w490) -> ("data"=w488:i8[], "no link"=w489:bool)  [unwired: 15 in, 2 out]
        n263 = case shown="False" w489 {
          tunnel: w488 -> [w495 _]
          tunnel: w487 -> [w494 _]
          frame False {
            n264 = Array Subset(array=w495, index=0, length=8) -> (w502:i8[])
            n265 = Array Subset(array=w495, index=8, length=8) -> (w498:i8[])
            n266 = Type Cast(type=0.0, x=w502) -> (*(type *) &x=w492:dbl)
            n267 = Type Cast(type=0.0, x=w498) -> (*(type *) &x=w491:dbl)
            n268 = Bundle(w492, w491) -> (w493:cluster{dbl, dbl})  [unwired: 1 in]
            n269 = Generate User Event(user event=w494, event data cluster=w493) -> ()  [unwired: 2 in, 2 out]
          }
          frame True {
          }
        }
      }
      frame True {
      }
    }
    "DIM Notifier loop" <- w478
  }
